vi "PerformCalibrationWithOptions.vi"(0 "MFCS_EZ":T4, 1 "Misselaneous Parameters":T3={"Ctr Odor Valve"=14, "Water Mix Valve"=12, "Total Odor Flow"=425.0, "Total Flow Setpoint"=531.25, "Control Pressure Channel"=1, "Mix Water Pressure Channel"=2} {"Water Mix Valve" items=["A1", "A2", "A3", "A4", "B1", "B2", "B3", "B4", "B5", "B6", "B7", "B8", "A5", "A6", "A7", "A8"]; "Ctr Odor Valve" items=["A1", "A2", "A3", "A4", "B1", "B2", "B3", "B4", "B5", "B6", "B7", "B8", "A5", "A6", "A7", "A8"]}, 2 "Mix Cluster":T5={"Ratio"=[0.6, 0.6, 0.6, 0.6, 0.6, 0.6, 0.6, 0.6], "Mix 2"=[8, 8, 8], "Mix 1"=[0, 0, 0]} {"Mix 1" items=["A1"=0, "A2"=1, "A3"=2, "A4"=3, "A5"=12]; "Mix 2" items=["B5"=8, "B6"=9, "B7"=10, "B8"=11, "A5"=12]}, 5 "Calibration Mode":T6(ring), 7 "Manual Default Set Pressures":dbl[](array[numeric])=[199.547, 665.1538332158755, 665.154, 665.154], 11 "Calibration Refs In":T2, 12 "Set Pressures In":dbl[][](array[numeric])=[[665.1538332158755, 622.4106177021335]], 13 "Ctr Pressure In":dbl=199.54651412930238) -> (4 "Ctr Pressure Out":dbl=199.54651412930238, 6 "Set Pressures Out":dbl[][](array[numeric])=[[665.1538332158755, 622.4106177021335]], 8 "Calibration Refs Out":T2, 10 "File Cluster":T1, 15 "Manual Default Set Pressures Out":dbl[](array[numeric])=[199.547, 665.1538332158755, 665.154, 665.154])   [LabVIEW 2016]
uses:
  <userlib>/Fluigent/Fluigent MFCS/FluigentMFCS_Full.llb/_EZmfcsRefNum.ctl
  <userlib>/Fluigent/Fluigent MFCS/FluigentMFCS_Full.llb/_EZmfcsEnum.ctl
  <userlib>/_OpenG.lib/array/array.llb/Index 1D Array Elements (String)__ogtk.vi
  <vilib>/Utility/file.llb/Write Delimited Spreadsheet (string).vi
panel:
  in  "Master Valves":u16(ring) items=["A1", "A2", "A3", "A4", "B1", "B2", "B3", "B4", "B5", "B6", "B7", "B8", "A5", "A6", "A7", "A8", ""]
  out "Pressure Group":u8[](array[numeric])=[3, 3, 3, 3, 4, 4, 4, 4]
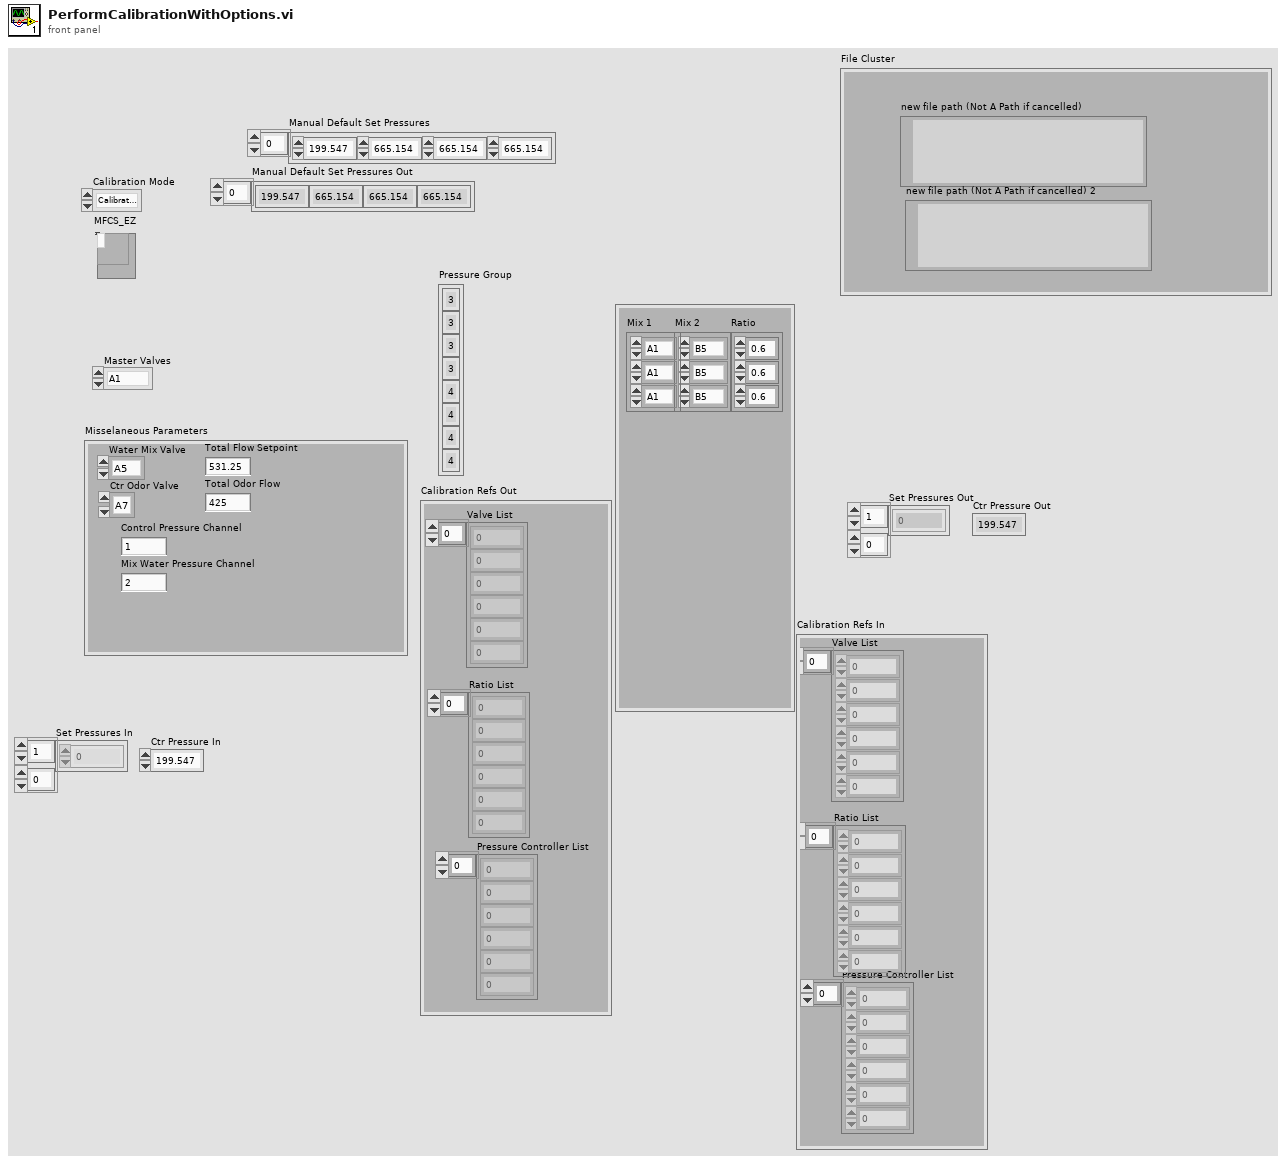
[diagram p1: front panel]
types:
  T1 = cluster{"new file path (Not A Path if cancelled)":path, "new file path (Not A Path if cancelled) 2":path}
  T2 = cluster{"Pressure Controller List":u8[], "Ratio List":dbl[], "Valve List":u16[]}
  T3 = cluster{"Ctr Odor Valve":u16, "Water Mix Valve":u16, "Total Odor Flow":dbl, "Total Flow Setpoint":dbl, "Control Pressure Channel":u16, "Mix Water Pressure Channel":u16}
  T4 = typedef "_EZmfcsRefNum.ctl" = refnum<k1>
  T5 = cluster{"Ratio":dbl[], "Mix 2":u16[], "Mix 1":u16[]}
  T6 = enum16{"Calibrate All", "Control Only", "Odors Only"}
  T7 = enum16{"nothing", "All + Keep Old", "All + Remove Old", "Nothing", "New Only", "Nothin3", "Nothing4", "Nothing5", "Cancel"}
  T8 = enum16{"Left Button", "Center Button", "Right Button", "Window Close"}
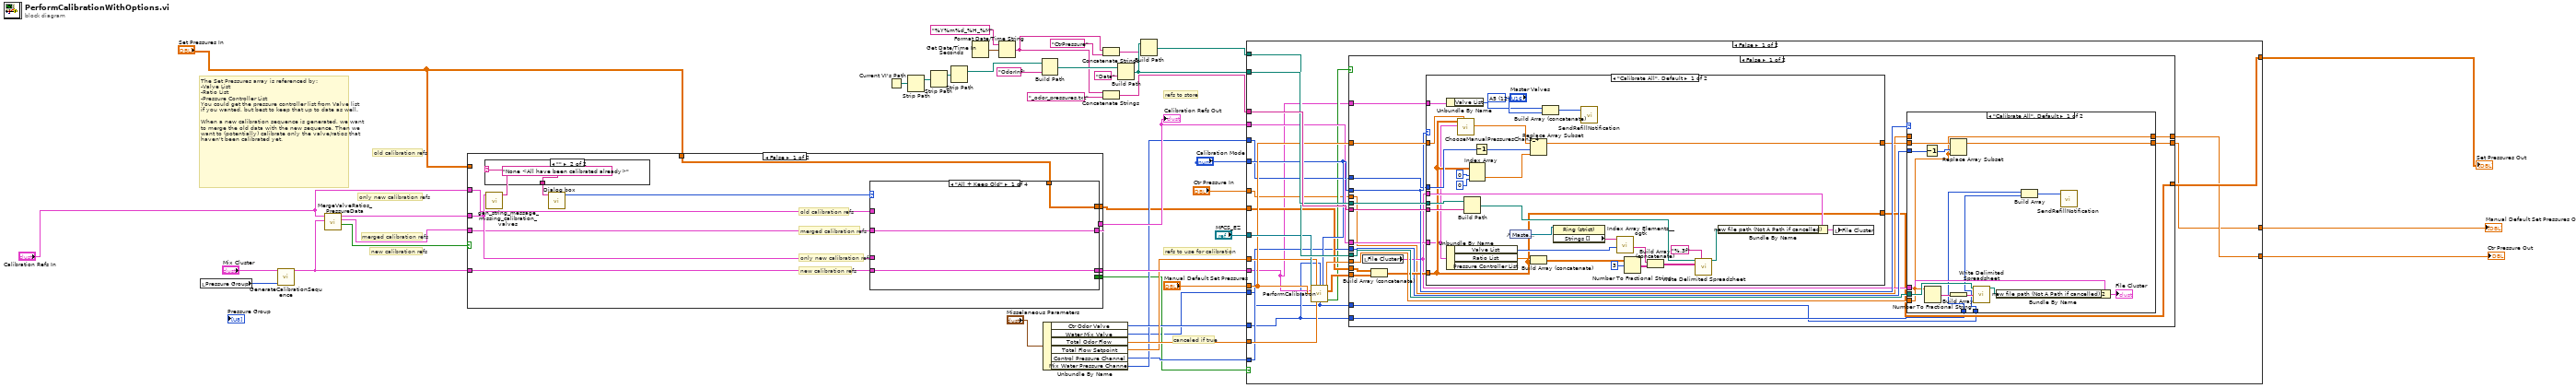
[diagram p0: block diagram]
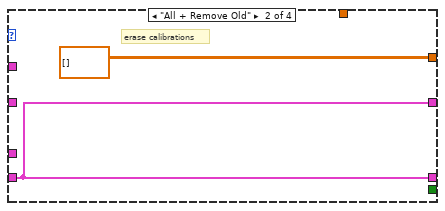
[diagram p7: hidden frame]
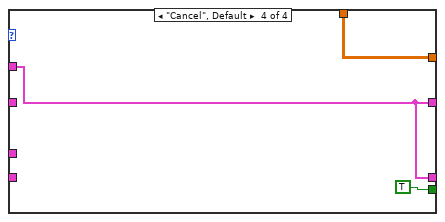
[diagram p9: hidden frame]
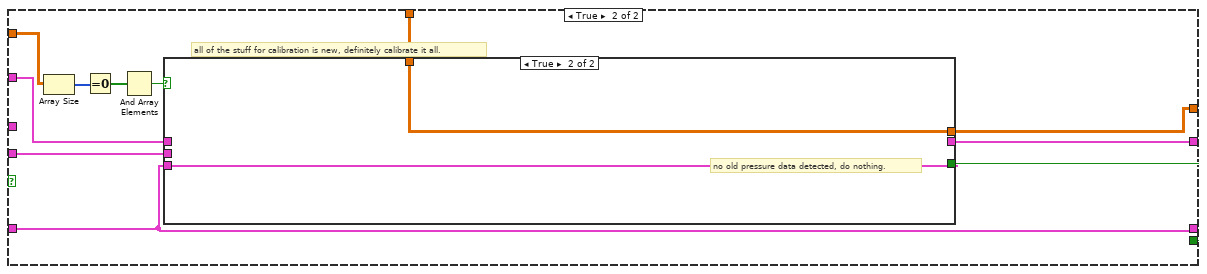
[diagram p10: hidden frame]
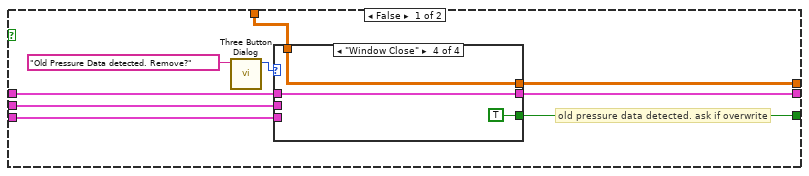
[diagram p11: hidden frame]
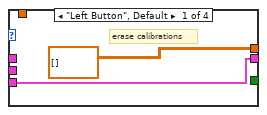
[diagram p12: hidden frame]
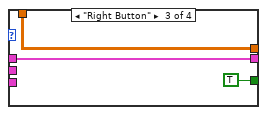
[diagram p14: hidden frame]
diagram:
  # "old calibration refs"
  # "merged calibration refs"
  # "new calibration refs"
  # "only new calibration refs"
  # "canceled if true"
  # "refs to store"
  # "refs to use for calibration"
  # "The Set Pressures array is referenced by:\n-Valve List\n-Ratio List\n-Pressure Controller List\nYou could get the pressure controller list from Valve list if you wanted, but best to keep that up to date as well.\n\nWhen a new calibration sequence is generated, we want to merge the old data with the new sequence. Then we want to (potentially) calibrate only the valve/ratios that haven't been calibrated yet."
  n1 = local read "Pressure Group"() -> (w30:u8[])
  n2 = call "GenerateCalibrationSequence.vi"("Pressure Group"=w30, "Mix Cluster"="Mix Cluster") -> ("Calibration Refs"=w22:T2)  [unwired: 9 in]
  n3 = call "MergeValveRatios_PressureData.vi"("New Calibration Refs"=w22, "Old Calibration Refs"="Calibration Refs In") -> ("None already calibrated?"=w24:bool, "Merged Calibration Refs"=w21:T2, "Only New Calibration Refs"=w23:T2)  [unwired: 7 in]
  n4 = case shown="False" w24 {
    tunnel: w23 -> [w52 _]
    tunnel: w22 -> [w53 w74]
    tunnel: w21 -> [w51 w72]
    tunnel: [w50 w73] -> w19
    tunnel: [w49 w74] -> w20
    tunnel: [w48 w75] -> w6
    tunnel: "Calibration Refs In" -> [w47 w71]
    tunnel: "Set Pressures In" -> [_ w70]
    tunnel: "Set Pressures In" -> [w44 w69]
    tunnel: [w43 w68] -> w2
    frame False {
      # "old calibration refs"
      # "merged calibration refs"
      # "new calibration refs"
      # "only new calibration refs"
      n5 = call "gen_string_message_missing_calibration_valves.vi"("Missing Calibration Refs"=w52) -> ("String"=w46:string)  [unwired: 9 in]
      n6 = case shown="\"\"" w46 {
        selector: w46 -> [w55 _]
        tunnel: [w55 "None <All have been calibrated already>"] -> w45
        frame "False", Default {
        }
        frame "" {
        }
      }
      n7 = call "Dialog box.vi"("Missing Str"=w45) -> ("Response"=w54:T7)  [unwired: 9 in]
      n8 = case shown="\"All + Keep Old\"" w54 {
        tunnel: w53 -> [w58 w61 _ _]
        tunnel: w52 -> [_ _ w64 _]
        tunnel: w51 -> [w59 _ w63 _]
        tunnel: [w59 w61 w63 w66] -> w50
        tunnel: [w58 w61 w64 w66] -> w49
        tunnel: [_ _ _ TRUE] -> w48
        tunnel: w47 -> [_ _ _ w66]
        tunnel: w44 -> [w57 _ w62 w65]
        tunnel: [w57 dbl[][] [] w62 w65] -> w43
        frame "All + Keep Old" {
        }
        frame "All + Remove Old" {
          # "erase calibrations"
        }
        frame "New Only" {
        }
        frame "Cancel", Default {
        }
      }
    }
    frame True {
      # "all of the stuff for calibration is new, definitely calibrate it all."
      n9 = Array Size(array=w70) -> (size(s)=w78:i32[])
      n10 = Equal To 0?(x=w78) -> (x = 0?=w77:bool[])
      n11 = And Array Elements(Boolean array=w77) -> (logical AND=w76:bool)
      n12 = case shown="True" w76 {
        tunnel: [w85 _] -> w75
        tunnel: w74 -> [w84 w99]
        tunnel: [w83 w99] -> w73
        tunnel: w72 -> [w82 _]
        tunnel: w71 -> [w81 _]
        tunnel: w69 -> [w80 w98]
        tunnel: [w79 w98] -> w68
        frame False {
          # "old pressure data detected. ask if overwrite"
          n13 = call <vilib>:"Three Button Dialog.vi"("message"="Old Pressure Data detected. Remove?") -> ("Which Button?"=w86:T8)  [unwired: 10 in]
          n14 = case shown="\"Window Close\"" w86 {
            tunnel: [_ _ TRUE TRUE] -> w85
            tunnel: w84 -> [w89 _ _ _]
            tunnel: [w89 w91 w93 w96] -> w83
            tunnel: w82 -> [_ w91 _ _]
            tunnel: w81 -> [_ _ w93 w96]
            tunnel: w80 -> [_ w90 w92 w95]
            tunnel: [dbl[][] [] w90 w92 w95] -> w79
            frame "Left Button", Default {
              # "erase calibrations"
            }
            frame "Center Button" {
              # "don't overwrite"
            }
            frame "Right Button" {
            }
            frame "Window Close" {
            }
          }
        }
        frame True {
          # "no old pressure data detected, do nothing."
        }
      }
    }
  }
  "Calibration Refs Out" <- w19
  n15 = Current VI's Path() -> (path=w5:path)
  n16 = Strip Path(path=w5) -> (stripped path=w4:path)  [unwired: 1 out]
  n17 = Strip Path(path=w4) -> (stripped path=w29:path)  [unwired: 1 out]
  n18 = Strip Path(path=w29) -> (stripped path=w28:path)  [unwired: 1 out]
  n19 = Get Date/Time In Seconds() -> (seconds since 1Jan1904=w41:timestamp)
  n20 = Format Date/Time String(time format string (%c)="%Y%m%d_%H_%M", seconds (now)=w41) -> (date/time string=w34:string)  [unwired: 1 in]
  n21 = Build Path(base path=w28, name or relative path="OdorInf") -> (appended path=w38:path)
  n22 = Unbundle By Name("Misselaneous Parameters") -> ("Ctr Odor Valve"=w14:u16, "Water Mix Valve"=w1:u16, "Total Odor Flow"=w16:dbl, "Total Flow Setpoint"=w15:dbl, "Control Pressure Channel"=w12:u16, "Mix Water Pressure Channel"=w13:u16)
  n23 = Concatenate Strings(w34, "CtrPressure" ("string")) -> (w32:string)
  n24 = Concatenate Strings(w34, "_odor_pressures.txt" ("string")) -> (w36:string)
  n25 = Build Path(base path=w38, name or relative path="Data") -> (appended path=w35:path)
  n26 = Build Path(base path=w35, name or relative path=w32) -> (appended path=w31:path)
  n27 = case shown="False" w6 {
    tunnel: w36 -> [w121 _]
    tunnel: w35 -> [w120 _]
    tunnel: w31 -> [w119 _]
    tunnel: "MFCS_EZ" -> [w118 _]
    tunnel: "Manual Default Set Pressures" -> [w116 w195]
    tunnel: "Calibration Mode" -> [w115 _]
    tunnel: w13 -> [w114 _]
    tunnel: w20 -> [w102 _]
    tunnel: w2 -> [w112 w194]
    tunnel: w19 -> [w111 _]
    tunnel: w1 -> [w100 _]
    tunnel: w16 -> [w110 _]
    tunnel: w15 -> [w109 _]
    tunnel: w14 -> [w101 _]
    tunnel: w12 -> [w108 _]
    tunnel: [w107 w194] -> w10
    tunnel: "Ctr Pressure In" -> [w103 w196]
    tunnel: [w106 w196] -> w8
    tunnel: [w105 w195] -> w7
    frame False {
      n28 = call "PerformCalibration.vi"("MFCS_EZ"=w118, "Total Flow Setpoint"=w109, "Ctr Water Valve"=w101, "Calibration Mode"=w115, "Calibration Refs"=w102, "Manual Default Set Pressures"=w116, "Total Odor Flow"=w110, "Water Mix Valve"=w100) -> ("Ctr Pressure"=w117:dbl, "Set Pressures"=w113:dbl[][], "Aborted?"=w104:bool)  [unwired: 5 in]
      n29 = case shown="False" w104 {
        tunnel: w121 -> [w142 _]
        tunnel: w120 -> [w141 _]
        tunnel: w119 -> [w140 _]
        tunnel: w117 -> [w139 _]
        tunnel: w116 -> [w138 w193]
        tunnel: w115 -> [w137 _]
        tunnel: w114 -> [w135 _]
        tunnel: w113 -> [w134 _]
        tunnel: w112 -> [w133 w191]
        tunnel: w111 -> [w131 _]
        tunnel: w108 -> [w130 _]
        tunnel: [w128 w191] -> w107
        tunnel: w103 -> [w127 w192]
        tunnel: [w126 w192] -> w106
        tunnel: [w125 w193] -> w105
        tunnel: w102 -> [w124 _]
        tunnel: w101 -> [w123 _]
        tunnel: w100 -> [w122 _]
        frame False {
          n30 = local read "File Cluster"() -> (w129:T1)
          n31 = Build Array (concatenate)(w133, w134) -> (w132:dbl[][])
          n32 = case shown="\"Calibrate All\", Default" w137 {
            tunnel: w142 -> [w170 _]
            tunnel: w141 -> [w168 _]
            tunnel: w132 -> [w148 w173]
            tunnel: w138 -> [w167 w174]
            tunnel: [w160 w174] -> w136
            tunnel: w135 -> [w163 _]
            tunnel: w131 -> [w147 _]
            tunnel: w129 -> [w149 _]
            tunnel: [w148 w173] -> w128
            tunnel: w124 -> [w146 _]
            frame "Calibrate All", Default {
              w145 = u16 12 items=["A1", "A2", "A3", "A4", "B1", "B2", "B3", "B4", "B5", "B6", "B7", "B8", "A5"] ("Master Valves")
              n33 = Unbundle By Name(w147) -> ("Valve List"=w159:u16[], "Ratio List"=w157:dbl[])  [unwired: 1 out]
              n34 = Unbundle By Name(w146) -> ("Valve List"=w144:u16[])
              n35 = call "ChooseManualPressuresChan3_4.vi"("Manual Pressure In"=w167, "Calibration Refs"=w147, "Set Pressures"=w148) -> ("Manual Pressure"=w164:dbl[])  [unwired: 8 in]
              n36 = Build Path(base path=w168, name or relative path=w170) -> (appended path=w169:path)
              n37 = Index Array(array=w148, index (row)=0, index (col)=0 ("disabled index (col)")) -> (element=w161:dbl)
              n38 = Decrement(x=w163) -> (x-1=w162:u16)
              n39 = control-ref of="Master Valves"() -> (w152:refnum<vi>)
              n40 = Replace Array Subset(array=w164, new element=w161, index=w162) -> (w160:dbl[])
              n41 = Build Array (concatenate)(w157, w148) -> (w156:dbl[][])
              n42 = Build Array (concatenate)(w144, w145) -> (w143:u16[])
              n43 = property on="Property Node" class="Ring (strict)"(reference=w152) -> ("Strings []"=w158:string[])  [unwired: 1 in, 2 out]
              n44 = call "SendRefillNotification.vi"("Valves IN"=w143) -> ()  [unwired: 11 in]
              n45 = call-poly <userlib>:"Index Array Elements__ogtk.vi"("indices"=w159, "array"=w158) -> ("elements"=w154:string[])  [unwired: 9 in]
              n46 = Number To Fractional String(number=w156, width (-)=i16 3) -> (F-format string=w155:string[][])  [unwired: 2 in]
              n47 = Build Array (concatenate)(w154, w155) -> (w153:string[][])
              n48 = call-poly <vilib>:"Write Delimited Spreadsheet.vi"("file path (dialog if empty)"=w169, "format (%s)"="%.3f" ("format (%.3f)"), "2D data"=w153) -> ("new file path (Not A Path if cancelled)"=w151:path)  [unwired: 11 in, 1 out]
              n49 = Bundle By Name(cluster=w149, "new file path (Not A Path if cancelled)"=w151) -> (w150:T1)
              n50 = local write "File Cluster"(w150) -> ()
            }
            frame "Control Only" {
            }
          }
          n51 = case shown="\"Calibrate All\", Default" w137 {
            tunnel: w140 -> [w188 _]
            tunnel: w139 -> [w178 _]
            tunnel: w136 -> [w185 w190]
            tunnel: w130 -> [w184 _]
            tunnel: [w182 w190] -> w125
            tunnel: w129 -> [w181 _]
            tunnel: w127 -> [_ w189]
            tunnel: [w178 w189] -> w126
            tunnel: w123 -> [w177 _]
            tunnel: w122 -> [w176 _]
            frame "Calibrate All", Default {
              n52 = Decrement(x=w184) -> (x-1=w183:u16)
              n53 = Number To Fractional String(number=w178) -> (F-format string=w187:string)  [unwired: 3 in]
              n54 = Replace Array Subset(array=w185, new element=w178, index=w183) -> (w182:dbl[])
              n55 = Build Array(w187) -> (w186:string[])
              n56 = call-poly <vilib>:"Write Delimited Spreadsheet.vi"("file path (dialog if empty)"=w188, "1D data"=w186) -> ("new file path (Not A Path if cancelled)"=w180:path)  [unwired: 12 in, 1 out]
              n57 = Bundle By Name(cluster=w181, "new file path (Not A Path if cancelled) 2"=w180) -> (→"File Cluster":T1)
              n58 = Build Array(w177, w176) -> (w175:u16[])
              n59 = call "SendRefillNotification.vi"("Valves IN"=w175) -> ()  [unwired: 11 in]
            }
            frame "Odors Only" {
            }
          }
        }
        frame True {
          # "PID aborted"
        }
      }
    }
    frame True {
      # "canceled"
    }
  }
  "Manual Default Set Pressures Out" <- w7
  "Set Pressures Out" <- w10
  "Ctr Pressure Out" <- w8
